vi "MSSQL_Delete.vi"(0 "connection reference":T1, 1 "表名":string, 2 "删除条件":string, 3 "异常输入":errorcluster) -> (6 "connection reference 2":T1, 7 "操作结果":bool, 9 "异常输出":errorcluster)   [LabVIEW 2018]
uses:
  <vilib>/addons/database/Connection.llb/Conn ObjectReference.ctl
  <vilib>/addons/database/Connection.llb/Conn Execute.vi
  <vilib>/addons/database/Recordset.llb/Rec Destroy - Connection.vi
  <vilib>/addons/database/NI_Database_API.lvlib
panel:
  # "Delete操作\ndelete from tbl_name where 列1 = ‘1’"
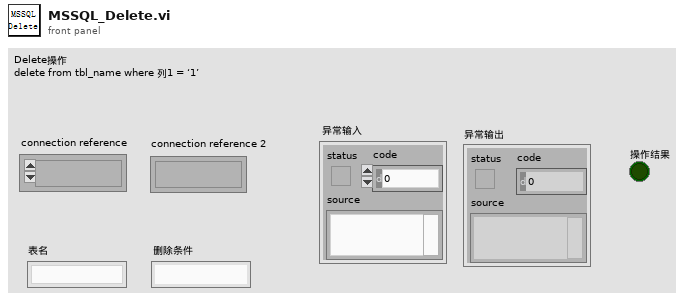
[diagram p1: front panel]
types:
  T1 = typedef "NI_Database_API.lvlib/Conn ObjectReference.ctl" = refnum<k1>
  T2 = typedef "NI_Database_API.lvlib/Rec ObjectReference.ctl" = refnum<k1>
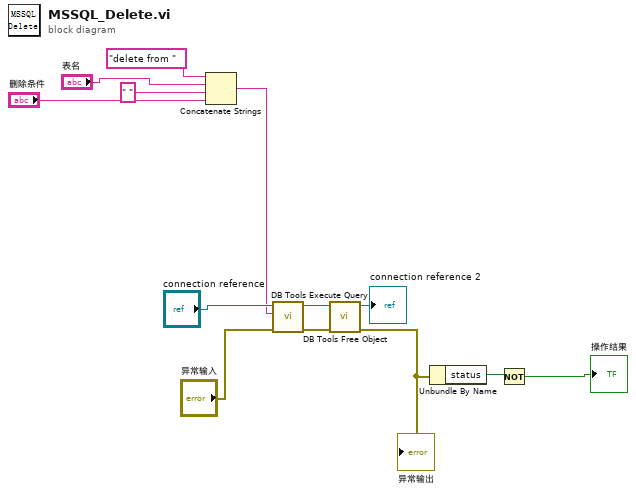
[diagram p0: block diagram]
diagram:
  n1 = Concatenate Strings("delete from ", "表名", " " ("字符串"), "删除条件") -> (w11:string)
  n2 = call-poly <vilib>:"DB Tools Execute Query.vi"("error in (no error)"="异常输入", "SQL query"=w11, "connection reference"="connection reference") -> ("error out"=w9:errorcluster, "recordset reference"=w10:T2)  [unwired: 5 in]
  n3 = call-poly <vilib>:"DB Tools Free Object.vi"("error in (no error)"=w9, "recordset reference"=w10) -> ("error out"=w6:errorcluster, "connection reference"=→"connection reference 2":T1)  [unwired: 8 in]
  "异常输出" <- w6
  n4 = Unbundle By Name(w6) -> ("status"=w4:bool)
  n5 = Not(x=w4) -> (.not. x?=→"操作结果":bool)
